vi "Do-Fft.vi"(11 "X":csg[](array[numeric])) -> (3 "FFT {X}":csg[](array[numeric]))   [LabVIEW 2015]
uses:
  <vilib>/Analysis/2dsp.llb/Complex FFT.vi
  <vilib>/Analysis/NI_AALPro.lvlib
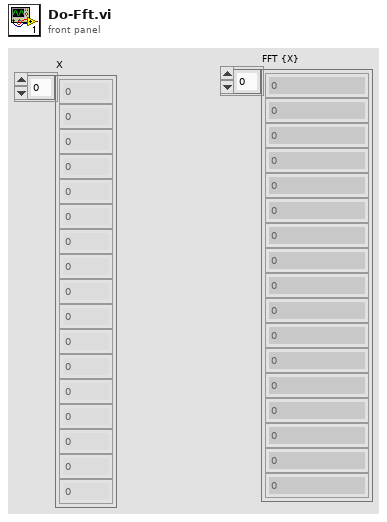
[diagram p1: front panel]
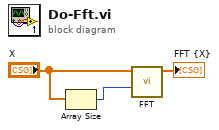
[diagram p0: block diagram]
diagram:
  n1 = Array Size(array="X") -> (size(s)=w1:i32)
  n2 = call-poly <vilib>:"FFT.vi"("FFT size"=w1, "X"="X") -> ("FFT {X}"=→"FFT {X}":cdb[])  [unwired: 8 in, 1 out]
